vi "XMLEASY.vi"(11 "Schedule Filename":string) -> (3 "output array":string[](array[string]))   [LabVIEW 2023]
uses:
  <vilib>/xml/Close Reference(Node).vi
  <vilib>/xml/NI_XML.lvlib
  <resource>/objmgr/DOMUserDefRef.rc
panel:
  out "output array 2":string[][](array[string])
  in  "error in (no error)":errorcluster
  out "error out":errorcluster
  out "XML":string
  out "Parse Errors":string
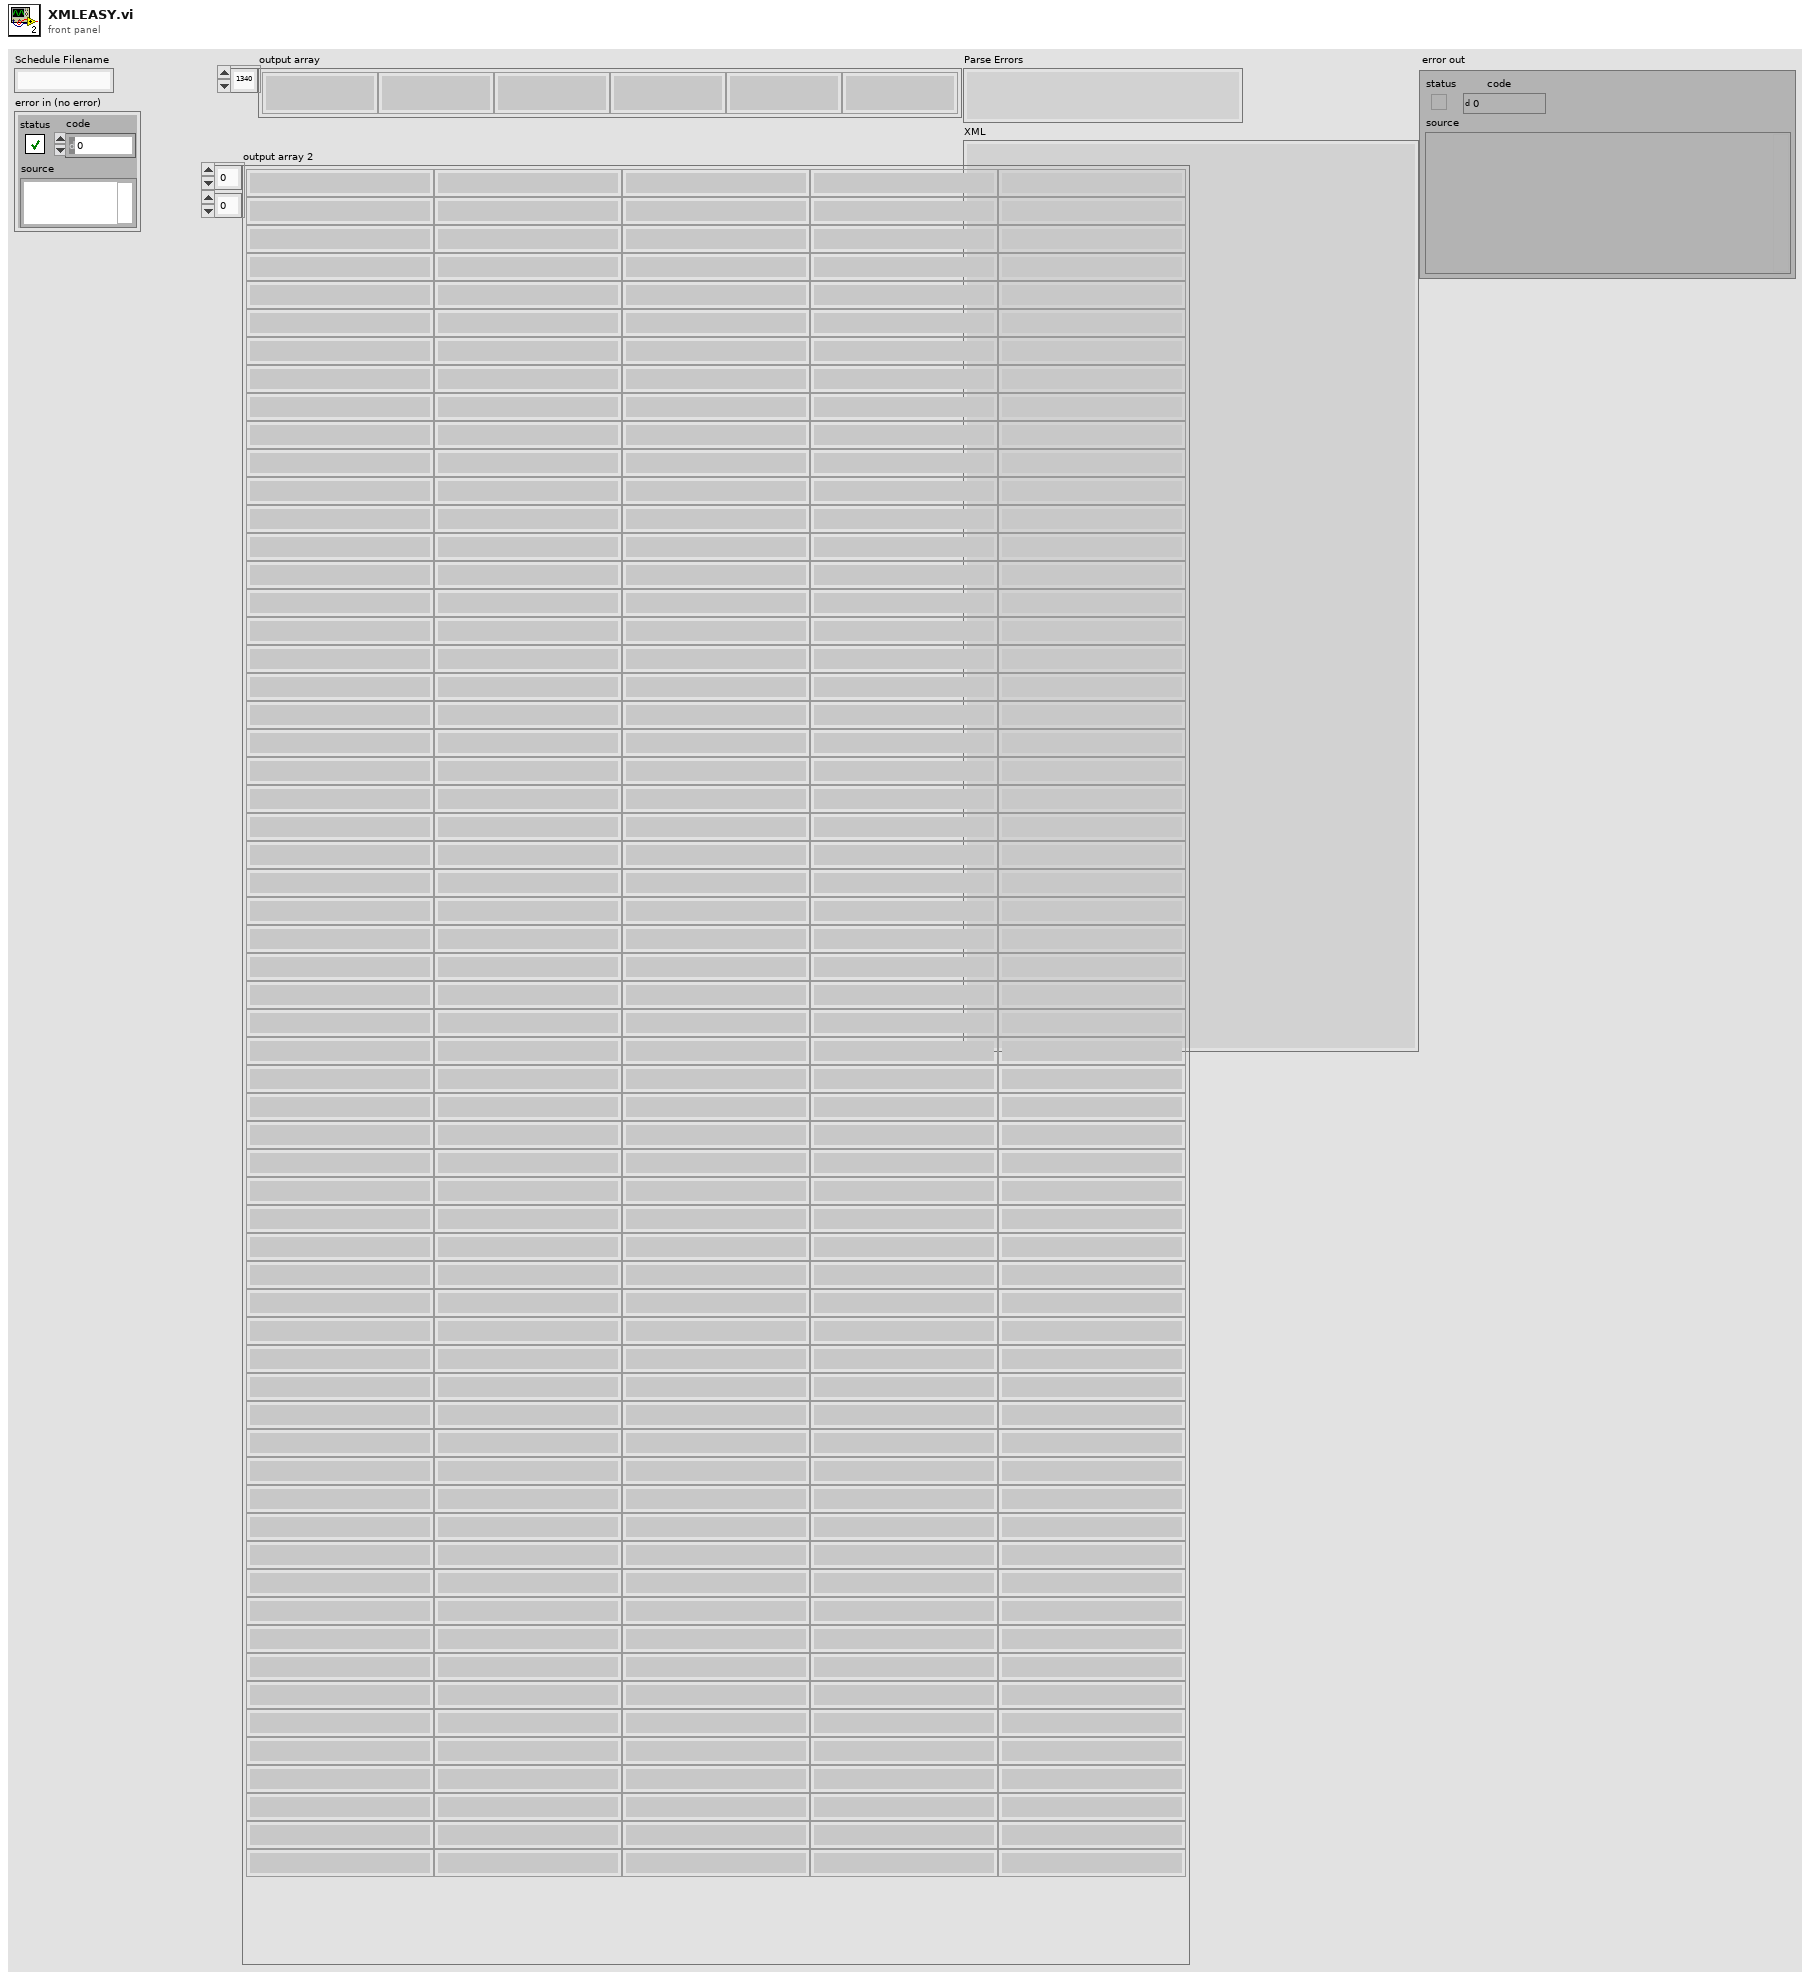
[diagram p1: front panel]
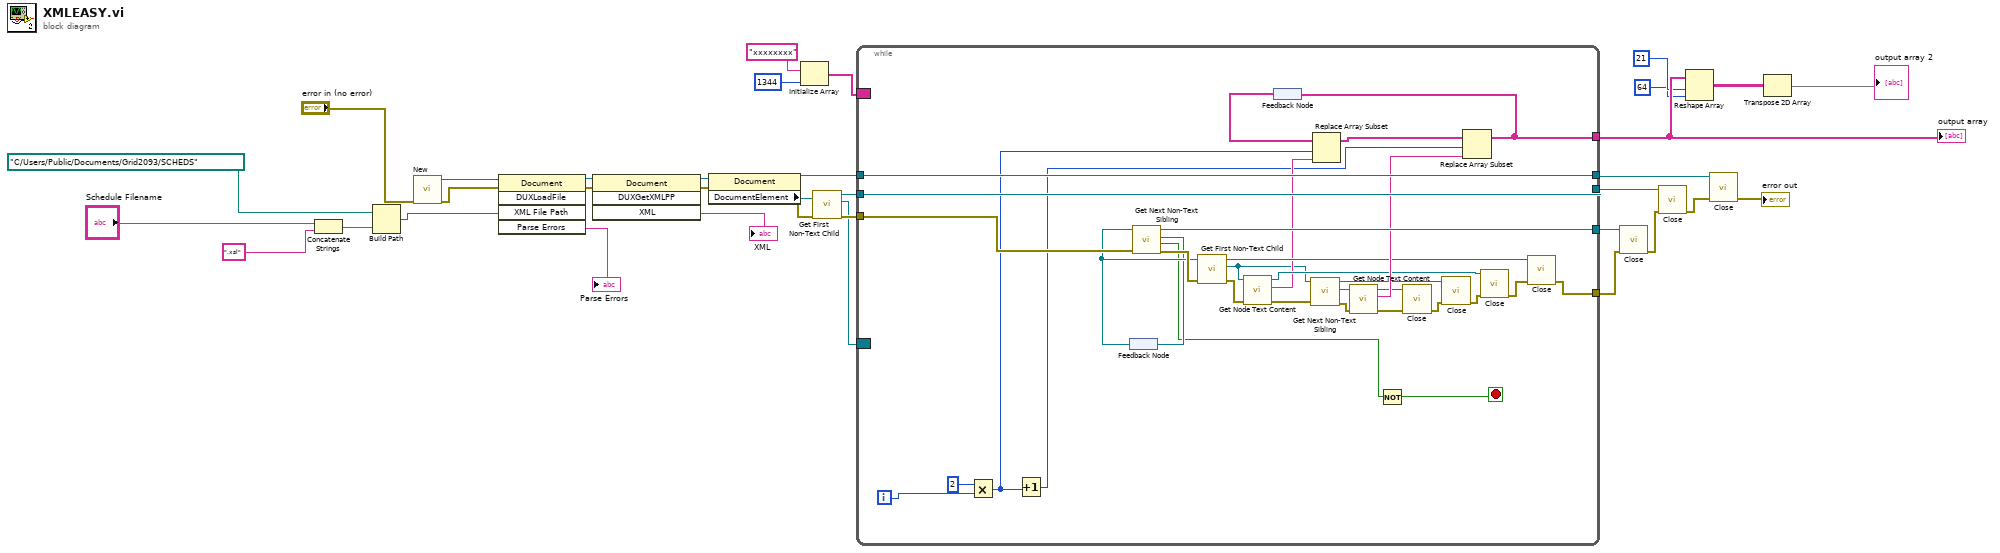
[diagram p0: block diagram]
diagram:
  n1 = Concatenate Strings("Schedule Filename", ".xsl" ("string")) -> (w26:string)
  n2 = Build Path(base path=path "C:/Users/Public/Documents/Grid2093/SCHEDS", name or relative path=w26) -> (appended path=w1:path)
  n3 = call <vilib>:"New.vi"("error in (no error)"="error in (no error)") -> ("error out"=w34:errorcluster, "DOM document out"=w35:refnum<k20>)  [unwired: 7 in]
  n4 = invoke class="Document" method="DUXLoadFile"(reference=w35, error in=w34, "XML File Path"=w1) -> (reference out=w33:refnum<k20>, error out=w32:errorcluster, "Parse Errors"=→"Parse Errors":string)  [unwired: 2 in, 2 out]
  n5 = invoke class="Document" method="DUXGetXMLPP"(reference=w33, error in=w32) -> (reference out=w31:refnum<k20>, error out=w30:errorcluster, "XML"=→"XML":string)  [unwired: 2 in, 1 out]
  n6 = property class="Document"(reference=w31, error in=w30) -> (reference out=w21:refnum<k20>, error out=w22:errorcluster, "DocumentElement"=w23:refnum<k20>)
  n7 = Initialize Array("xxxxxxxx", 1344 ("dimension size")) -> (w5:string[])
  n8 = call <vilib>:"Get First Non-Text Child.vi"("error in (no error)"=w22, "node in"=w23) -> ("error out"=w17:errorcluster, "child node"=w9:refnum<k20>, "node out"=w18:refnum<k20>)  [unwired: 6 in, 1 out]
  n9 = while {
    tunnel: w21 -> [w66]
    tunnel: w17 -> [w67]
    tunnel: w18 -> [w65]
    tunnel: [w66] -> w16
    tunnel: [w65] -> w15
    tunnel: [w64] -> w8
    tunnel: [w37] -> w11
    tunnel: [w63] -> w12
    border: w9 -> [_]
    border: w5 -> [_]
    i -> [w41]
    stop <- w46 stop-if-true
    n10 = Multiply(x=2, y=w41) -> (x*y=w39:i32)
    n11 = Increment(x=w39) -> (x+1=w38:i32)
    n12 = feedback #1() -> (w53:refnum<k20>)
    n13 = call <vilib>:"Get Next Non-Text Sibling.vi"("error in (no error)"=w67, "node in"=w53) -> ("error out"=w54:errorcluster, "found sibling node?"=w45:bool, "sibling node"=w47:refnum<k20>, "node out"=w63:refnum<k20>)  [unwired: 6 in]
    n14 = feedback-in #1(w47) -> ()
    n15 = call <vilib>:"Get First Non-Text Child.vi"("error in (no error)"=w54, "node in"=w53) -> ("error out"=w50:errorcluster, "child node"=w36:refnum<k20>, "node out"=w51:refnum<k20>)  [unwired: 6 in, 1 out]
    n16 = call <vilib>:"Get Node Text Content.vi"("error in (no error)"=w50, "node in"=w36) -> ("error out"=w48:errorcluster, "node text"=w42:string, "node out"=w49:refnum<k20>)  [unwired: 7 in]
    n17 = feedback #2() -> (w44:string[])
    n18 = call <vilib>:"Get Next Non-Text Sibling.vi"("error in (no error)"=w48, "node in"=w36) -> ("error out"=w58:errorcluster, "sibling node"=w59:refnum<k20>, "node out"=w57:refnum<k20>)  [unwired: 6 in, 1 out]
    n19 = Replace Array Subset(array=w44, new element=w42, index=w39) -> (w43:string[])
    n20 = call <vilib>:"Get Node Text Content.vi"("error in (no error)"=w58, "node in"=w59) -> ("error out"=w61:errorcluster, "node text"=w62:string, "node out"=w60:refnum<k20>)  [unwired: 7 in]
    n21 = Not(x=w45) -> (.not. x?=w46:bool)
    n22 = call-poly <vilib>:"Close.vi"("error in (no error)"=w61, "node"=w60) -> ("error out"=w56:errorcluster)  [unwired: 7 in]
    n23 = call-poly <vilib>:"Close.vi"("error in (no error)"=w56, "node"=w57) -> ("error out"=w55:errorcluster)  [unwired: 7 in]
    n24 = Replace Array Subset(array=w43, new element=w62, index=w38) -> (w64:string[])
    n25 = feedback-in #2(w64) -> ()
    n26 = call-poly <vilib>:"Close.vi"("error in (no error)"=w55, "node"=w49) -> ("error out"=w52:errorcluster)  [unwired: 7 in]
    n27 = call-poly <vilib>:"Close.vi"("error in (no error)"=w52, "node"=w51) -> ("error out"=w37:errorcluster)  [unwired: 7 in]
  }
  "output array" <- w8
  n28 = call-poly <vilib>:"Close.vi"("error in (no error)"=w11, "node"=w12) -> ("error out"=w13:errorcluster)  [unwired: 7 in]
  n29 = call-poly <vilib>:"Close.vi"("error in (no error)"=w13, "node"=w15) -> ("error out"=w14:errorcluster)  [unwired: 7 in]
  n30 = Reshape Array(w8, 21 ("dimension size"), 64 ("dimension size")) -> (w4:string[][])
  n31 = call-poly <vilib>:"Close.vi"("error in (no error)"=w14, "node"=w16) -> ("error out"=→"error out":errorcluster)  [unwired: 7 in]
  n32 = Transpose 2D Array(2D array=w4) -> (transposed array=→"output array 2":string[][])
